vi "Read Active Module.vi"(8 "error in":errorcluster, 11 "3300 in":refnum<class "3300.lvclass">) -> (0 "error out":errorcluster, 2 "Active Module":T1, 3 "3300 out":refnum<class "3300.lvclass">)   [LabVIEW 2019, in "3300.lvlib" / "3300.lvclass"]
uses:
  Library/3300.lvclass
  C:/Users/Public/Documents/Development/builds/Instruments/Electronic Load.lvlibp/Library/Electronic Load.lvclass
  Custom Controls/Modules.ctl
  Library/3300.lvclass/3300.ctl
  Accessors/Read Installed Modules.vi
  builds/Instruments/Electronic Load.lvlibp/Accessors/Read Active Channel.vi
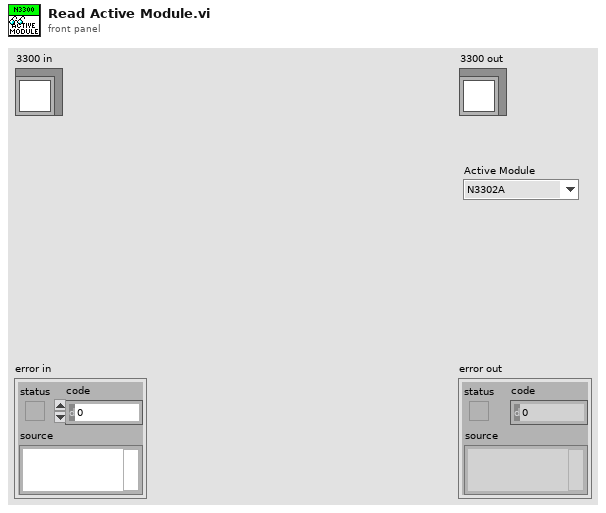
[diagram p1: front panel]
types:
  T1 = typedef "3300.lvlib/3300.lvclass/Modules.ctl" = enum16{"N3302A", "N3303A", "N3304A", "N3305A", "N3306A", "N3307A"}
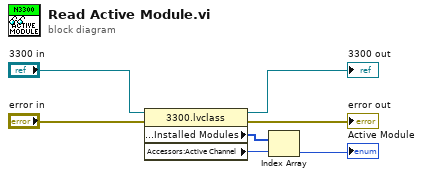
[diagram p0: block diagram]
diagram:
  n1 = property class="3300.lvclass"(reference="3300 in", error in="error in") -> (reference out=→"3300 out":refnum<class "3300.lvclass">, error out=→"error out":errorcluster, "Private:Accessors:Installed Modules"=w6:T1[], "Accessors:Active Channel"=w5:u32)
  n2 = Index Array(array=w6, index=w5) -> (element=→"Active Module":T1)
